vi "Send(Sub).vi"(7 "보내기":T1={"국번"="0", "커맨드"="81", "데이터 No."="00", "데이터"="1EA5"}, 10 "VISA 참조 번호 입력":refnum<visa-resource-name>) -> (0 "x = y?":bool, 3 "VISA 참조 번호 출력":refnum<visa-resource-name>)   [LabVIEW 2014]
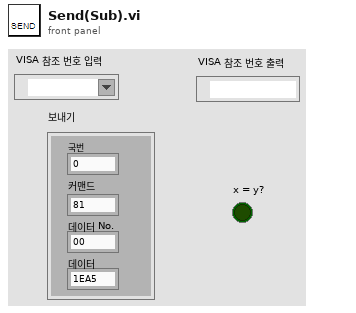
[diagram p1: front panel]
types:
  T1 = cluster{"국번":string, "커맨드":string, "데이터 No.":string, "데이터":string}
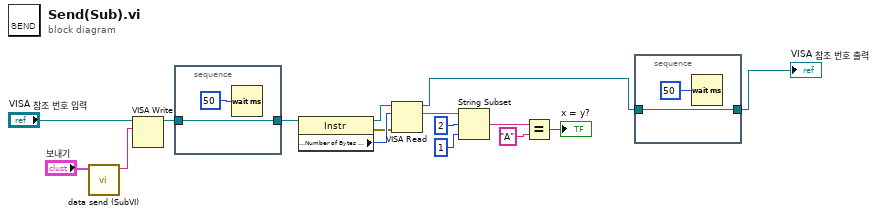
[diagram p0: block diagram]
diagram:
  n1 = call "data send (SubVI).vi"("보내기"="보내기") -> ("문자열"=w4:string)  [unwired: 10 in]
  n2 = VISA Write(VISA resource name="VISA 참조 번호 입력", write buffer=w4) -> (VISA resource name out=w10:refnum<visa-resource-name>)  [unwired: 1 in, 2 out]
  n3 = stacked-sequence {
    tunnel: w10 -> [w18]
    tunnel: [w18] -> w6
    frame #0 {
      n4 = Wait (ms)(milliseconds to wait=u32 50 ("delay before read (ms)")) -> ()  [unwired: 1 out]
    }
  }
  n5 = property on="Property Node" class="Instr"(reference=w6) -> (reference out=w7:refnum<visa-resource-name>, error out=w8:errorcluster, "Serial Settings:Number of Bytes at Serial Port"=w9:u32)  [unwired: 1 in]
  n6 = VISA Read(VISA resource name=w7, byte count=w9, error in (no error)=w8) -> (VISA resource name out=w2:refnum<visa-resource-name>, read buffer=w13:string)  [unwired: 2 out]
  n7 = String Subset(string=w13, offset (0)=2 ("오프셋(0)"), length (rest)=1 ("길이(나머지)")) -> (substring=w14:string)
  n8 = Equal?(x=w14, y="A") -> (x = y?=→"x = y?":bool)
  n9 = stacked-sequence {
    tunnel: w2 -> [w20]
    tunnel: [w20] -> w1
    frame #0 {
      n10 = Wait (ms)(milliseconds to wait=u32 50 ("delay before read (ms)")) -> ()  [unwired: 1 out]
    }
  }
  "VISA 참조 번호 출력" <- w1
